vi "Load All Firmware Config Data.vi"(8 "Error In":errorcluster) -> (0 "Error Out":errorcluster, 1 "Firmwares":T2[][][](array[typedef]), 2 "Devices":T1[][](array[typedef]), 3 "Families":string[](array[string]))   [LabVIEW 2011, in "LVH-LINX.lvlib"]
uses:
  LVH-LINX.lvlib
  Type Defs/Device Firmware.ctl
  Type Defs/Device Data.ctl
  Type Defs/All Firmware Data FGV States.ctl
  <vilib>/LabVIEW Hacker/LVH-Toolbox/Common/LVH-Common.lvlib
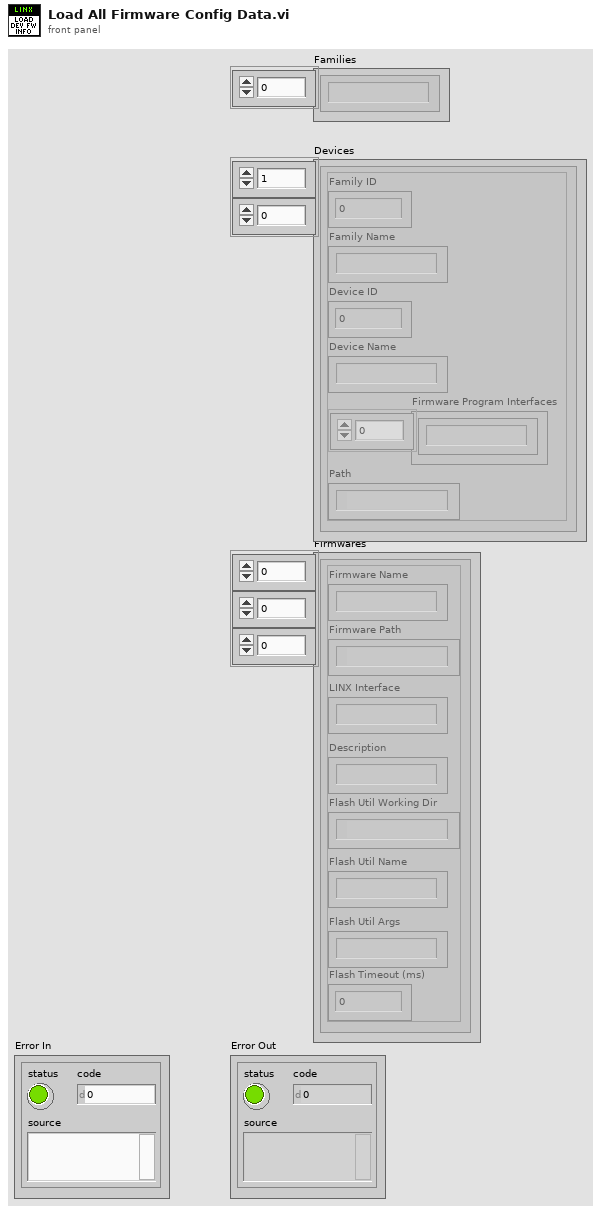
[diagram p1: front panel]
types:
  T1 = typedef "LVH-LINX.lvlib/Device Data.ctl" = cluster{"Family ID":i32, "Family Name":string, "Device ID":i32, "Device Name":string, "Firmware Program Interfaces":string[], "Path":path}
  T2 = typedef "LVH-LINX.lvlib/Device Firmware.ctl" = cluster{"Firmware Name":string, "Firmware Path":path, "Description":string, "LINX Interface":string, "Flash Util Working Dir":path, "Flash Util Name":string, "Flash Util Args":string, "Flash Timeout (ms)":i32}
  T3 = typedef "LVH-LINX.lvlib/All Firmware Data FGV States.ctl" = enum16{"Set", "Get"}
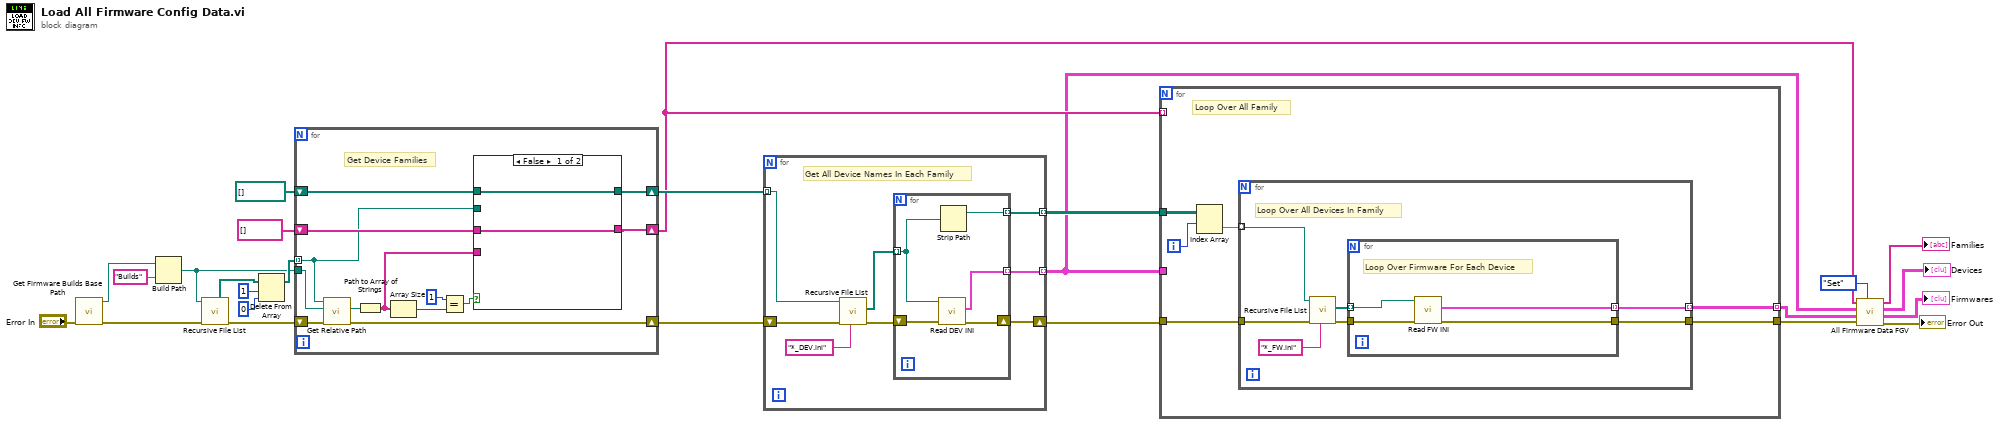
[diagram p0: block diagram]
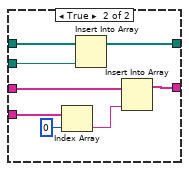
[diagram p2: hidden frame]
diagram:
  n1 = call "Get Firmware Builds Base Path.vi"("Error In"="Error In") -> ("Error Out"=w24:errorcluster, "Firmware Builds Base Path"=w3:path)  [unwired: 9 in]
  n2 = Build Path(base path=w3, name or relative path="Builds") -> (appended path=w1:path)
  n3 = call <vilib>:"Recursive File List.vi"("error in (no error)"=w24, "Folder Path"=w1) -> ("error out"=w23:errorcluster, "All Folders"=w20:path[])  [unwired: 5 in, 3 out]
  n4 = Delete From Array(array=w20, length=1 ("index"), index=0) -> (array with subset deleted=w19:path[])  [unwired: 1 out]
  n5 = for {
    tunnel: w19 -> [w28] mode=indexing
    tunnel: w1 -> [w29]
    shift-right: [w31] -> w9
    shift-left: string[] [] -> [w30]
    shift-right: [w37] -> w15
    shift-left: w23 -> [w38]
    shift-right: [w27] -> w16
    shift-left: path[] [] -> [w26]
    # "Get Device Families"
    n6 = call <vilib>:"Get Relative Path.vi"("Error In"=w38, "Relative Path Root"=w29, "File / Folder"=w28) -> ("Error Out"=w37:errorcluster, "Relative Path"=w36:path)  [unwired: 6 in, 1 out]
    n7 = Path to Array of Strings(0:w36) -> (2:w32:string[])  [unwired: 1 out]
    n8 = Array Size(array=w32) -> (size(s)=w35:i32)
    n9 = Equal?(x=1, y=w35) -> (x = y?=w33:bool)
    n10 = case shown="False" w33 {
      tunnel: w32 -> [_ w48]
      tunnel: [w40 w45] -> w31
      tunnel: w30 -> [w40 w46]
      tunnel: w28 -> [_ w42]
      tunnel: [w39 w43] -> w27
      tunnel: w26 -> [w39 w41]
      frame False {
      }
      frame True {
        n11 = Index Array(array=w48, index=0) -> (element=w44:string)
        n12 = Insert Into Array(array=w41, new element=w42) -> (w43:path[])  [unwired: 1 in]
        n13 = Insert Into Array(array=w46, new element=w44) -> (w45:string[])  [unwired: 1 in]
      }
    }
  }
  n14 = for {
    tunnel: w16 -> [w56] mode=indexing
    tunnel: [w51] -> w7 mode=indexing
    shift-right: [w50] -> w14
    shift-left: w15 -> [w55]
    tunnel: [w49] -> w13 mode=indexing
    # "Get All Device Names In Each Family"
    n15 = call <vilib>:"Recursive File List.vi"("pattern"="*_DEV.ini", "error in (no error)"=w55, "Folder Path"=w56) -> ("error out"=w52:errorcluster, "All Files in Dir"=w53:path[])  [unwired: 4 in, 3 out]
    n16 = for {
      tunnel: w53 -> [w58] mode=indexing
      tunnel: [w57] -> w51 mode=indexing
      shift-right: [w59] -> w50
      shift-left: w52 -> [w60]
      tunnel: [w61] -> w49 mode=indexing
      n17 = call "Read DEV INI.vi"("Error In"=w60, "Firmware INI Path"=w58) -> ("Error Out"=w59:errorcluster, "Device Data"=w57:T1)  [unwired: 7 in, 1 out]
      n18 = Strip Path(path=w58) -> (stripped path=w61:path)  [unwired: 1 out]
    }
  }
  n19 = for {
    tunnel: w7 -> [_]
    tunnel: [w66] -> w10 mode=indexing
    tunnel: w14 -> [w62]
    tunnel: [w65] -> w12
    tunnel: w13 -> [w63]
    tunnel: w9 -> [_] mode=indexing
    i -> [w67]
    # "Loop Over All Family"
    n20 = Index Array(array=w63, index (row)=w67) -> (element=w64:path[])  [unwired: 1 in]
    n21 = for {
      tunnel: [w73] -> w66 mode=indexing
      tunnel: [w74] -> w65
      tunnel: w64 -> [w70] mode=indexing
      tunnel: w62 -> [w71]
      # "Loop Over All Devices In Family"
      n22 = call <vilib>:"Recursive File List.vi"("pattern"="*_FW.ini", "error in (no error)"=w71, "Folder Path"=w70) -> ("error out"=w68:errorcluster, "All Files in Dir"=w69:path[])  [unwired: 4 in, 3 out]
      n23 = for {
        tunnel: [w78] -> w74
        tunnel: [w77] -> w73 mode=indexing
        tunnel: w69 -> [w76] mode=indexing
        tunnel: w68 -> [w75]
        # "Loop Over Firmware For Each Device"
        n24 = call "Read FW INI.vi"("Error In"=w75, "Firmware INI Path"=w76) -> ("Error Out"=w78:errorcluster, "Firmware Config"=w77:T2)  [unwired: 7 in, 1 out]
      }
    }
  }
  n25 = call "All Firmware Data FGV.vi"("All Firmware Data FGV States"=All_Firmware_Data_FGV_States."Set", "Error In"=w12, "Firmwares"=w10, "Devices"=w7, "Families"=w9) -> ("Error Out"=→"Error Out":errorcluster, "Firmwares"=→"Firmwares":T2[][][], "Devices"=→"Devices":T1[][], "Families"=→"Families":string[])  [unwired: 3 in]
